vi "LWXPS_ZygoAmplitudeGet.vi"(0 "XPS Reference IN":refnum<k24>, 11 "LabVIEW error IN":errorcluster) -> (3 "XPS Reference OUT":refnum<k24>, 4 "Returned error code":i32, 6 "Zygo reference signal status":i32, 8 "Measuring channel amplitude 1":i32, 10 "Measuring channel amplitude 2":i32, 14 "LabVIEW error OUT":errorcluster, 15 "XPS Error String":string)   [LabVIEW 2014]
uses:
  D:/XPSQ8_LabView_Library/Development/Source/Dll/Newport.XPS.CommandInterface.dll
  Dll/Newport.XPS.CommandInterface.dll
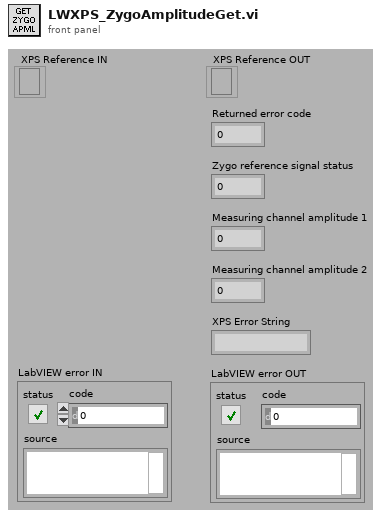
[diagram p1: front panel]
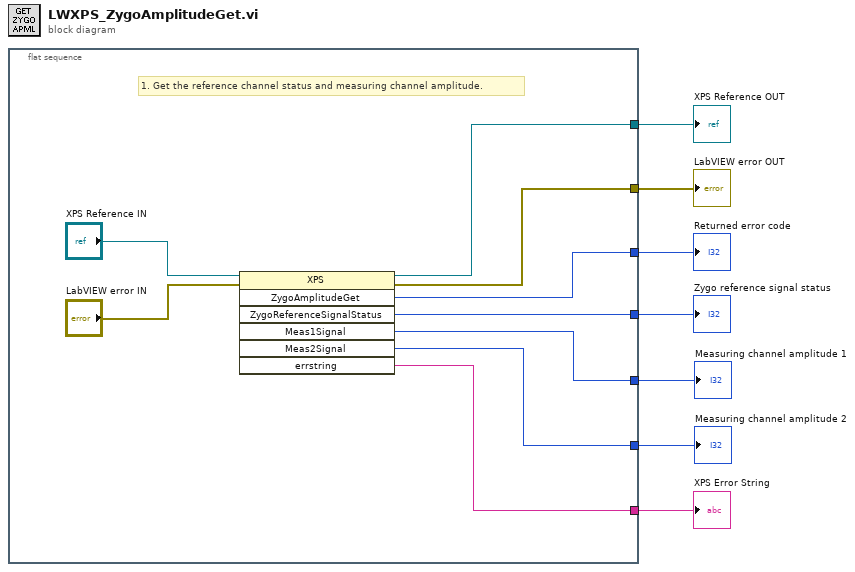
[diagram p0: block diagram]
diagram:
  n1 = flat-sequence {
    tunnel: [w14] -> w7
    tunnel: [w12] -> w6
    tunnel: [w15] -> w5
    tunnel: [w10] -> w2
    tunnel: [w11] -> w1
    tunnel: [w9] -> w4
    tunnel: [w8] -> w3
    frame #0 {
      # "1. Get the reference channel status and measuring channel amplitude."
      n2 = invoke class="XPS" method="ZygoAmplitudeGet"(reference="XPS Reference IN", error in="LabVIEW error IN") -> (reference out=w14:refnum<k24>, error out=w12:errorcluster, "ZygoAmplitudeGet"=w15:i32, "ZygoReferenceSignalStatus"=w8:i32, "Meas1Signal"=w10:i32, "Meas2Signal"=w11:i32, "errstring"=w9:string)  [unwired: 5 in]
    }
  }
  "XPS Error String" <- w4
  "XPS Reference OUT" <- w7
  "LabVIEW error OUT" <- w6
  "Returned error code" <- w5
  "Zygo reference signal status" <- w3
  "Measuring channel amplitude 1" <- w2
  "Measuring channel amplitude 2" <- w1
